vi "Test Sum.vi"(11 "Error in":errorcluster) -> (15 "Error out":errorcluster)   [LabVIEW 2020, in "SumOfFactorialsTests.lvlib"]
doc: "This VI validates sum of factorials"
uses:
  SumOfFactorialsTests.lvlib
  <vilib>/addons/_JKI Toolkits/Caraya/classes/Test Suite/Define Test Suite (JUnit Report).vi
  <vilib>/SLL Drona/APIs/Stimulus/ControlValue/SetValueAuto.vi
  <vilib>/SLL Drona/APIs/Assert/AssertControlValue/AlmostEqual.vi
  <vilib>/SLL Drona/APIs/Stimulus/VI/CloseVI.vi
  <vilib>/Utility/error.llb/Error Cluster From Error Code.vi
  <vilib>/ErrorRing/Error Ring.xnode
  <vilib>/addons/_JKI Toolkits/Caraya/classes/Test Suite/Test Suite.lvclass
  <vilib>/addons/_JKI Toolkits/Caraya/classes/Test/Test.lvclass
  <vilib>/SLL Drona/Drona.lvlib
  <vilib>/Wiresmith Technology/G CLI/CLI Class/CLI.lvclass
  <vilib>/SLL Drona/APIs/Stimulus/ControlValue/ControlValue.lvlib
  <vilib>/SLL Drona/APIs/Assert/AssertControlValue/AssertControlValue.lvlib
  <vilib>/SLL Drona/APIs/Stimulus/VI/VI.lvlib
panel:
  # "SUM OF FACTORIALS TEST"
  # "Test Trial"
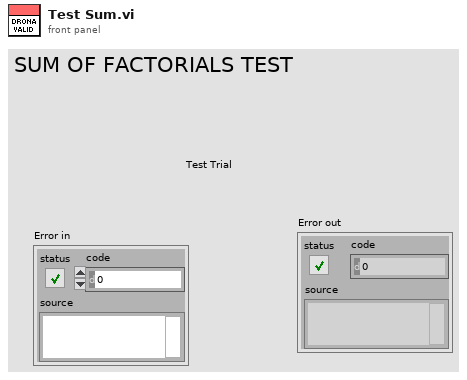
[diagram p1: front panel]
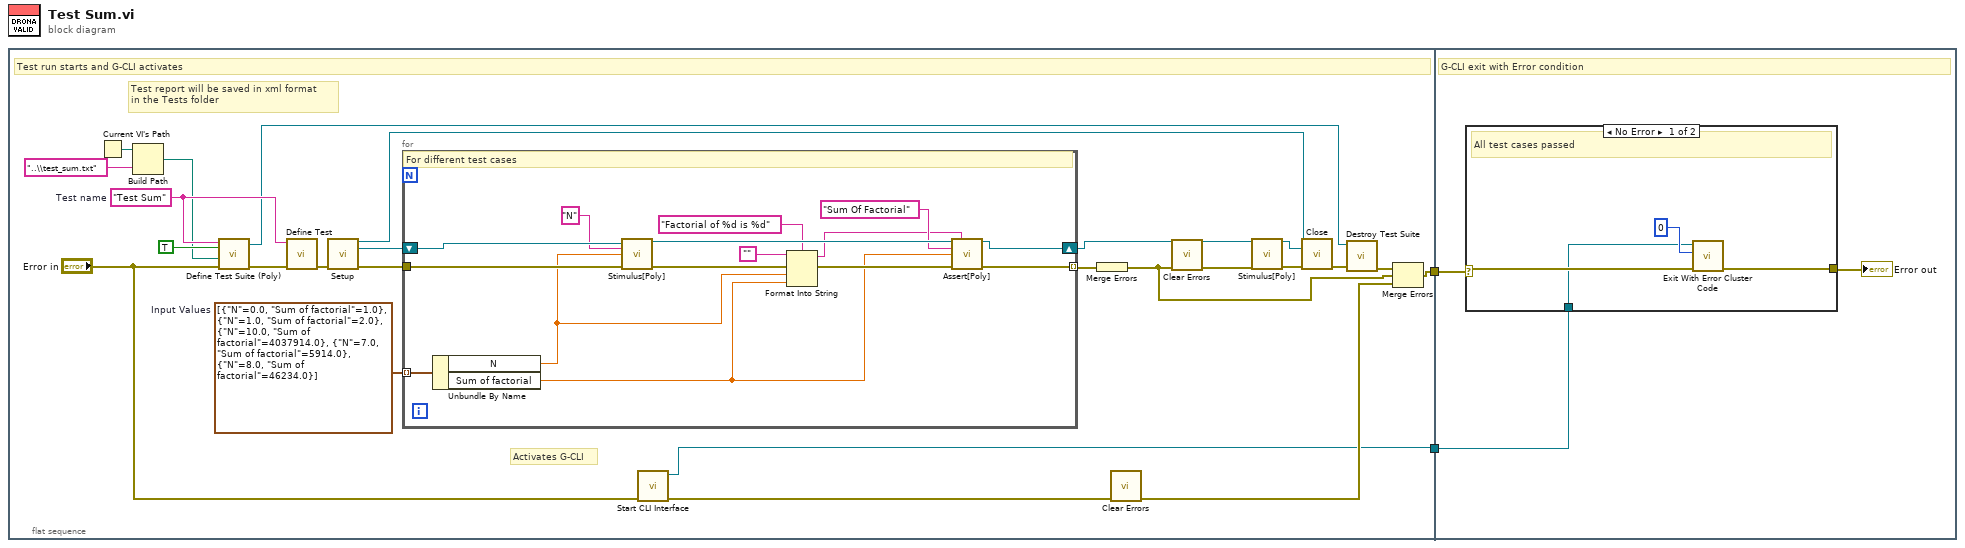
[diagram p0: block diagram]
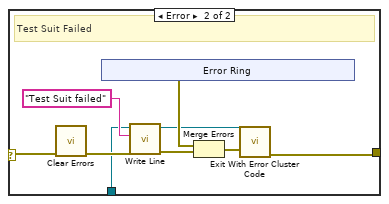
[diagram p2: hidden frame]
diagram:
  n1 = flat-sequence {
    tunnel: [w18] -> w2
    tunnel: [w15] -> w1
    tunnel: w2 -> [w45]
    tunnel: w1 -> [w43]
    frame #0 {
      w25 = cluster{"N":dbl, "Sum of factorial":dbl}[] [{"N"=0.0, "Sum of factorial"=1.0}, {"N"=1.0, "Sum of factorial"=2.0}, {"N"=10.0, "Sum of factorial"=4037914.0}, {"N"=7.0, "Sum of factorial"=5914.0}, {"N"=8.0, "Sum of factorial"=46234.0}]  # Input Values
      w12 = "Test Sum"  # Test name
      # "Test report will be saved in xml format\nin the Tests folder"
      # "Activates G-CLI"
      # "Test run starts and G-CLI activates"
      n2 = Current VI's Path() -> (path=w10:path)
      n3 = Build Path(base path=w10, name or relative path="..\\test_sum.txt") -> (appended path=w8:path)
      n4 = call-poly <vilib>:"Define Test Suite (Poly).vi"("error in (no error)"="Error in", "Report Path"=w8, "Interactive"=TRUE, "Label (VI Title)"=w12) -> ("error out"=w14:errorcluster, "Test Suite"=w5:refnum<class "Test Suite.lvclass">)  [unwired: 6 in]
      n5 = call <vilib>:"Define Test.vi"("error in (no error)"=w14, "Label (VI Title)"=w12) -> ("error out"=w27:errorcluster)  [unwired: 9 in]
      n6 = call <vilib>:"Setup.vi"("error in"=w27) -> ("Application Ref"=w23:refnum<vi>, "VI Reference Out"=w24:refnum<vi>, "error out"=w26:errorcluster)  [unwired: 12 in]
      n7 = for {
        tunnel: w25 -> [w39] mode=indexing
        shift-right: [w29] -> w22
        shift-left: w24 -> [w38]
        tunnel: w26 -> [w41]
        tunnel: [w42] -> w19 mode=indexing
        # "For different test cases"
        n8 = Unbundle By Name(w39) -> ("N"=w32:dbl, "Sum of factorial"=w28:dbl)
        n9 = call-poly <vilib>:"Stimulus[Poly].vi"("VI Reference In"=w38, "Control Path"="N", "Value (Signaling)"=w32, "error in"=w41) -> ("VI Reference Out"=w36:refnum<vi>, "error out"=w40:errorcluster)  [unwired: 10 in]
        n10 = Format Into String(format string="Factorial of %d is %d", initial string="", error in=w40, w32, w28) -> (resulting string=w30:string, error out=w35:errorcluster)
        n11 = call-poly <vilib>:"Assert[Poly].vi"("VI Reference In"=w36, "Test Label"=w30, "Control Path"="Sum Of Factorial", "Control Value"=w28, "Error In"=w35) -> ("VI Reference Out"=w29:refnum<vi>, "Error Out"=w42:errorcluster)  [unwired: 9 in]
      }
      n12 = call <vilib>:"Start CLI Interface.vi"("error in (no error)"="Error in") -> ("error out"=w16:errorcluster, "CLI out"=w15:refnum<class "CLI.lvclass">)  [unwired: 7 in, 2 out]
      n13 = Merge Errors(w19) -> (w3:errorcluster)
      n14 = call <vilib>:"Clear Errors.vi"("error in (no error)"=w16) -> ("error out"=w17:errorcluster)  [unwired: 5 in, 1 out]
      n15 = call <vilib>:"Clear Errors.vi"("error in (no error)"=w3) -> ("error out"=w4:errorcluster)  [unwired: 5 in, 1 out]
      n16 = call-poly <vilib>:"Stimulus[Poly].vi"("VI Reference In"=w22, "error in"=w4) -> ("VI Reference Out"=w21:refnum<vi>, "error out"=w20:errorcluster)  [unwired: 12 in]
      n17 = call <vilib>:"Close.vi"("Application Ref"=w23, "VI Reference"=w21, "error in"=w20) -> ("error out"=w7:errorcluster)  [unwired: 12 in]
      n18 = call-dynamic "Destroy Test Suite.vi"("error in (no error)"=w7, "Test Suite in"=w5) -> ("error out"=w6:errorcluster)  [unwired: 8 in, 1 out]
      n19 = Merge Errors(w6, w3, w17) -> (w18:errorcluster)
    }
    frame #1 {
      # "G-CLI exit with Error condition"
      n20 = case shown="No Error" w45 {
        selector: w45 -> [w49 w56]
        tunnel: [w48 w58] -> w44
        tunnel: w43 -> [w46 w51]
        frame No Error {
          # "All test cases passed"
          n21 = call <vilib>:"Exit With Error Cluster Code.vi"("error in (no error)"=w49, "No Error Code (0)"=0, "CLI in"=w46) -> ("error out"=w48:errorcluster)  [unwired: 8 in]
        }
        frame Error {
          # "Test Suit Failed"
          n22 = call <vilib>:"Clear Errors.vi"("error in (no error)"=w56) -> ("error out"=w55:errorcluster)  [unwired: 5 in, 1 out]
          n23 = xnode "Error Ring"() -> ("error out"=w53:errorcluster)
          n24 = call <vilib>:"Write Line.vi"("error in (no error)"=w55, "Text to Write"="Test Suit failed", "CLI in"=w51) -> ("error out"=w52:errorcluster, "CLI out"=w50:refnum<class "CLI.lvclass">)  [unwired: 7 in]
          n25 = Merge Errors(w53, w52) -> (w54:errorcluster)
          n26 = call <vilib>:"Exit With Error Cluster Code.vi"("error in (no error)"=w54, "CLI in"=w50) -> ("error out"=w58:errorcluster)  [unwired: 9 in]
        }
      }
      "Error out" <- w44
    }
  }
